vi "Recall Load.vi"(0 "LV MDI in":refnum<class "LV MDI.lvclass">, 11 "error in (no error)":errorcluster) -> (4 "LV MDI out":refnum<class "LV MDI.lvclass">, 8 "Name[]":string[](array[string]), 15 "error out":errorcluster)   [LabVIEW 2016, in "LV MDI.lvclass"]
uses:
  LV MDI.lvclass
  Document/Document.lvclass
  LV MDI.lvclass/LV MDI.ctl
  Document/Document.lvclass/Document.ctl
  Document/Child Classes/LV Doc/Child Classes/LV DEV/Public/Instantiate with Path.vi
  Document/Child Classes/LV Doc/Child Classes/LV DEV/LV DEV.lvclass
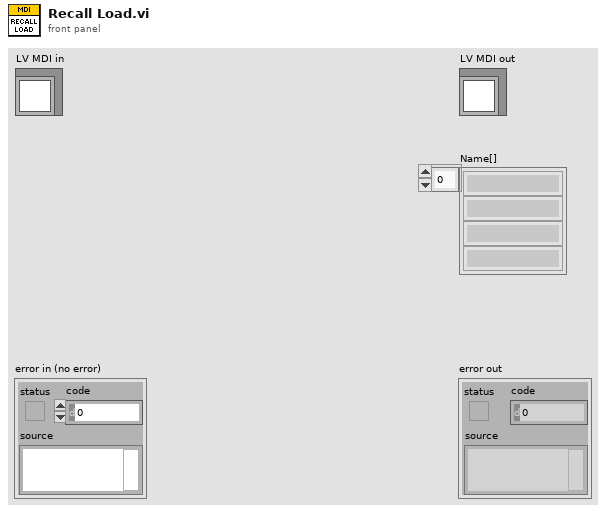
[diagram p1: front panel]
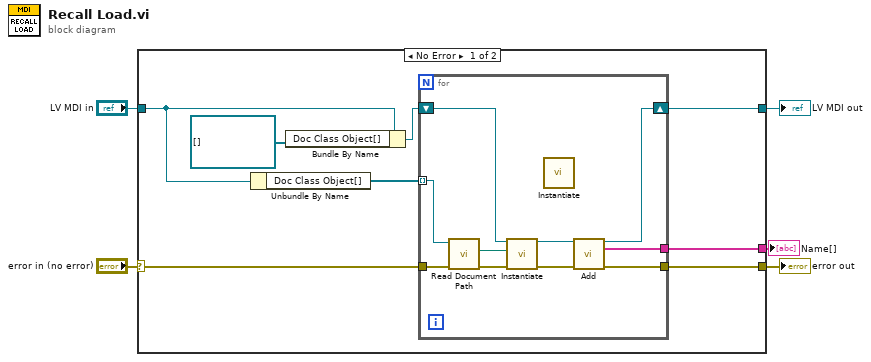
[diagram p0: block diagram]
diagram:
  n1 = case shown="No Error" "error in (no error)" {
    selector: "error in (no error)" -> [w13 w25]
    tunnel: [w12 w25] -> w4
    tunnel: [w10 w24] -> w2
    tunnel: "LV MDI in" -> [w8 w24]
    tunnel: [w9 _] -> w1
    frame No Error {
      n2 = Unbundle By Name(w8) -> ("Doc Class Object[]"=w11:refnum<class "Document.lvclass">[])
      n3 = Bundle By Name(cluster=w8, "Doc Class Object[]"=refnum<class "Document.lvclass">[] []) -> (w7:refnum<class "LV MDI.lvclass">)
      n4 = for {
        tunnel: w13 -> [w23]
        tunnel: [w22] -> w12
        tunnel: w11 -> [w14] mode=indexing
        tunnel: [w15] -> w9
        shift-right: [w21] -> w10
        shift-left: w7 -> [w20]
        n5 = call "Read Document Path.vi"("error in (no error)"=w23, "Document in"=w14) -> ("error out"=w18:errorcluster, "Document Path"=w16:path)  [unwired: 7 in, 1 out]
        n6 = call "Instantiate.vi"("LV MDI.lvclass"=w20, "Document Path"=w16, "Error in"=w18) -> ("LV MDI.lvclass"=w19:refnum<class "LV MDI.lvclass">, "Error Out"=w17:errorcluster)  [unwired: 11 in]
        n7 = call-poly "Instantiate.vi"() -> ()  [unwired: 14 in, 2 out]
        n8 = call "Add.vi"("LV MDI.lvclass"=w19, "error in (no error)"=w17) -> ("LV MDI.lvclass"=w21:refnum<class "LV MDI.lvclass">, "Name[]"=w15:string[], "error out"=w22:errorcluster)  [unwired: 11 in]
      }
    }
    frame Error {
    }
  }
  "error out" <- w4
  "LV MDI out" <- w2
  "Name[]" <- w1
